vi "Close Sessions.vi"(11 "Semiconductor Module Context":T1) -> (0 "error out":errorcluster)   [LabVIEW 2013]
uses:
  <vilib>/NI_TestStand_SemiconductorModule/NI_TestStand_Semiconductor_Module.lvlibp/PinMap/General/SemiconductorModuleContext.ctl
  <vilib>/NI_TestStand_SemiconductorModule/NI_TestStand_Semiconductor_Module.lvlibp
  Instruments/VNA/Pin Map API/VNA Custom Instrument.lvlib
  Instruments/DMM/Pin Map API/DMM Custom Instruments.lvlib
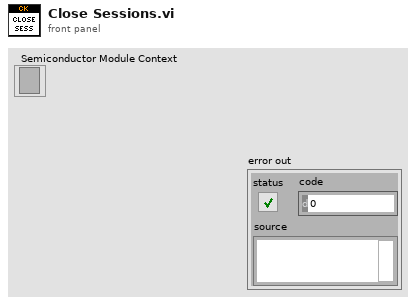
[diagram p1: front panel]
types:
  T1 = typedef "NI_TestStand_Semiconductor_Module.lvlibp/SemiconductorModuleContext.ctl" = refnum<k7>
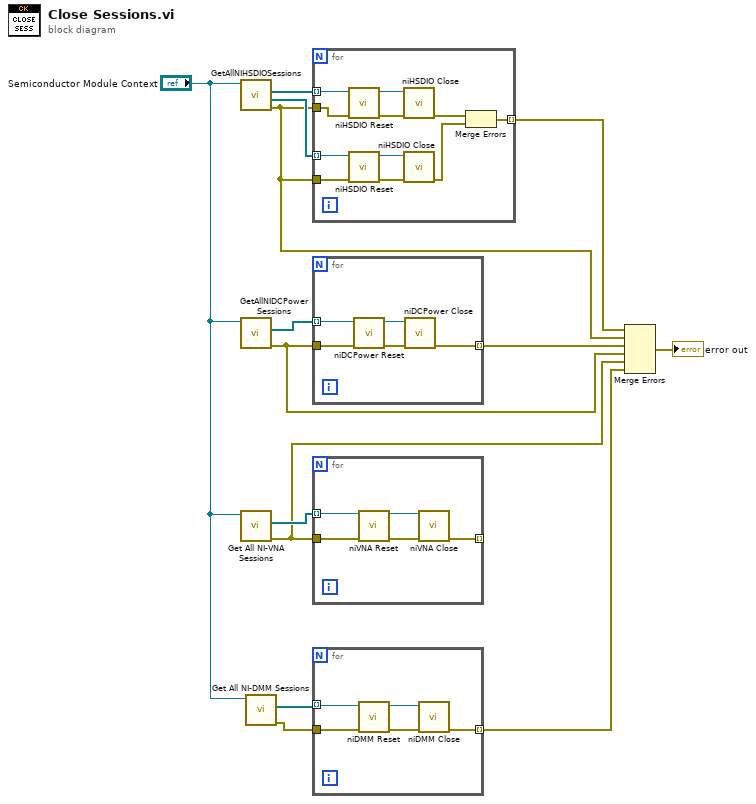
[diagram p0: block diagram]
diagram:
  n1 = call <vilib>:"GetAllNIHSDIOSessions.vi"("Semiconductor Module Context"="Semiconductor Module Context") -> ("error out"=w8:errorcluster, "Generation Sessions"=w13:refnum<k15>[], "Acquisition Sessions"=w14:refnum<k15>[])  [unwired: 7 in, 1 out]
  n2 = call <vilib>:"GetAllNIDCPowerSessions.vi"("Semiconductor Module Context"="Semiconductor Module Context") -> ("error out"=w6:errorcluster, "Instrument Sessions"=w12:refnum<k15>[])  [unwired: 8 in, 1 out]
  n3 = call "Get All NI-VNA Sessions.vi"("Semiconductor Module Context"="Semiconductor Module Context") -> ("error out"=w5:errorcluster, "Instrument Sessions"=w11:refnum<k15>[])  [unwired: 8 in, 1 out]
  n4 = call "Get All NI-DMM Sessions.vi"("Semiconductor Module Context"="Semiconductor Module Context") -> ("error out"=w3:errorcluster, "Instrument Sessions"=w4:refnum<k15>[])  [unwired: 8 in, 1 out]
  n5 = for {
    tunnel: w8 -> [w22]
    tunnel: w14 -> [w21] mode=indexing
    tunnel: w13 -> [w18] mode=indexing
    tunnel: w8 -> [w19]
    tunnel: [w15] -> w9 mode=indexing
    n6 = call <instrlib>:"niHSDIO Reset.vi"("error in (no error)"=w22, "instrument handle"=w21) -> ("error out"=w23:errorcluster, "instrument handle out"=w20:refnum<k15>)  [unwired: 8 in]
    n7 = call <instrlib>:"niHSDIO Reset.vi"("error in (no error)"=w19, "instrument handle"=w18) -> ("error out"=w25:errorcluster, "instrument handle out"=w24:refnum<k15>)  [unwired: 8 in]
    n8 = call <instrlib>:"niHSDIO Close.vi"("error in (no error)"=w23, "instrument handle"=w20) -> ("error out"=w17:errorcluster)  [unwired: 9 in]
    n9 = call <instrlib>:"niHSDIO Close.vi"("error in (no error)"=w25, "instrument handle"=w24) -> ("error out"=w16:errorcluster)  [unwired: 9 in]
    n10 = Merge Errors(w17, w16) -> (w15:errorcluster)
  }
  n11 = for {
    tunnel: w6 -> [w29]
    tunnel: w12 -> [w28] mode=indexing
    tunnel: [w30] -> w7 mode=indexing
    n12 = call <instrlib>:"niDCPower Reset.vi"("error in (no error)"=w29, "instrument handle"=w28) -> ("error out"=w26:errorcluster, "instrument handle out"=w27:refnum<k15>)  [unwired: 8 in]
    n13 = call <instrlib>:"niDCPower Close.vi"("error in (no error)"=w26, "instrument handle"=w27) -> ("error out"=w30:errorcluster)  [unwired: 9 in]
  }
  n14 = for {
    tunnel: w5 -> [w35]
    tunnel: w11 -> [w34] mode=indexing
    tunnel: [w31] -> _ mode=indexing
    n15 = call <instrlib>:"niVNA Reset.vi"("instrument handle"=w34, "error in"=w35) -> ("instrument handle out"=w32:refnum<k15>, "error out"=w33:errorcluster)  [unwired: 12 in]
    n16 = call <instrlib>:"niVNA Close.vi"("instrument handle"=w32, "error in"=w33) -> ("error out"=w31:errorcluster)  [unwired: 13 in]
  }
  n17 = for {
    tunnel: w3 -> [w40]
    tunnel: w4 -> [w36] mode=indexing
    tunnel: [w37] -> w2 mode=indexing
    n18 = call <instrlib>:"niDMM Reset.vi"("error in (no error)"=w40, "instrument handle"=w36) -> ("error out"=w39:errorcluster, "instrument handle out"=w38:refnum<k15>)  [unwired: 8 in]
    n19 = call <instrlib>:"niDMM Close.vi"("error in (no error)"=w39, "instrument handle"=w38) -> ("error out"=w37:errorcluster)  [unwired: 9 in]
  }
  n20 = Merge Errors(w9, w8, w7, w6, w5, w2) -> (→"error out":errorcluster)
